vi "Save Document.vi"(8 "error in (no error)":errorcluster, 10 "Path":path, 11 "Document in":refnum<k20>) -> (0 "error out":errorcluster, 3 "Document out":refnum<k20>)   [LabVIEW 2013, in "JUnit XML.lvlib"]
doc: "Saves the document to a file."
uses:
  JUnit XML.lvlib
  <resource>/objmgr/DOMUserDefRef.rc
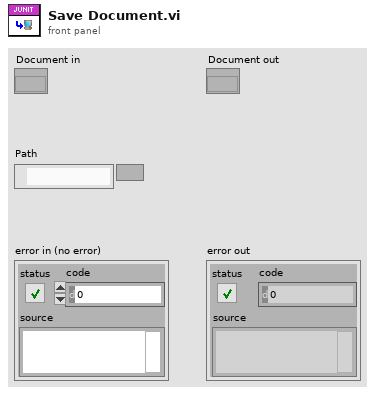
[diagram p1: front panel]
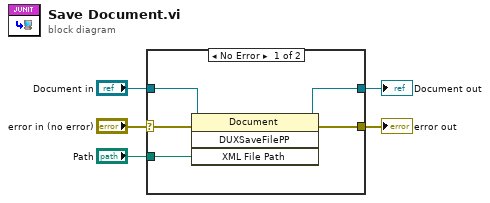
[diagram p0: block diagram]
diagram:
  n1 = case shown="No Error" "error in (no error)" {
    selector: "error in (no error)" -> [w6 w12]
    tunnel: [w10 w12] -> w5
    tunnel: "Path" -> [w9 _]
    tunnel: "Document in" -> [w8 w11]
    tunnel: [w7 w11] -> w2
    frame No Error {
      n2 = invoke class="Document" method="DUXSaveFilePP"(reference=w8, error in=w6, "XML File Path"=w9) -> (reference out=w7:refnum<k20>, error out=w10:errorcluster)  [unwired: 1 in, 2 out]
    }
    frame Error {
    }
  }
  "Document out" <- w2
  "error out" <- w5
